vi "practice 4.vi"() -> ()   [LabVIEW 2018]
panel:
  out "文字列 8":string
  out "文字列 7":string
  out "数値 3":dbl
  in  "クラスタ":cluster{"数値":dbl, "数値 2":dbl}
  out "数値 2":dbl
  in  "文字列 6":string
  out "文字列 5":string
  in  "文字列 4":string
  out "文字列 3":string
  in  "文字列 2":string
  in  "文字列":string
  out "数値":dbl
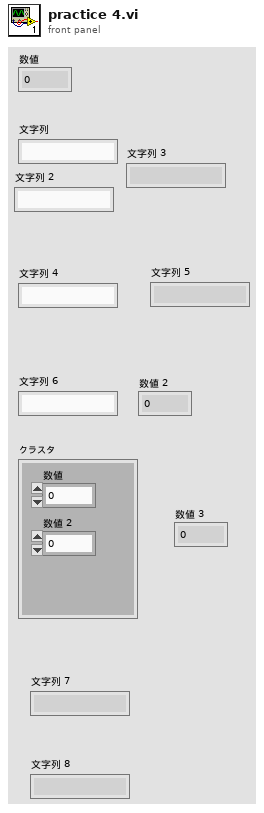
[diagram p1: front panel]
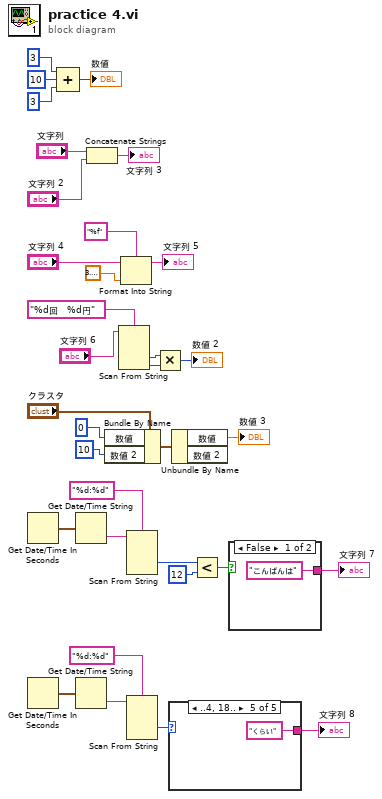
[diagram p0: block diagram]
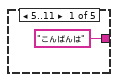
[diagram p2: hidden frame]
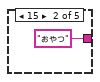
[diagram p3: hidden frame]
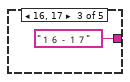
[diagram p4: hidden frame]
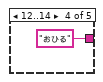
[diagram p5: hidden frame]
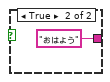
[diagram p6: hidden frame]
diagram:
  n1 = Get Date/Time In Seconds() -> (seconds since 1Jan1904=w12:timestamp)
  n2 = Get Date/Time In Seconds() -> (seconds since 1Jan1904=w3:timestamp)
  n3 = Compound Arithmetic op=unknown ("複合演算")(3, 10, 3) -> (→"数値":i32)
  n4 = Get Date/Time String(seconds (now)=w12) -> (time string=w6:string)  [unwired: 2 in, 1 out]
  n5 = Get Date/Time String(seconds (now)=w3) -> (time string=w5:string)  [unwired: 2 in, 1 out]
  n6 = Concatenate Strings("文字列", "文字列 2") -> (→"文字列 3":string)
  n7 = Bundle By Name(cluster="クラスタ", "数値"=0, "数値 2"=10) -> (w16:cluster{"数値":dbl, "数値 2":dbl})
  n8 = Scan From String(format string="%d回　%d円" ("形式文字列"), input string="文字列 6") -> (output 1=w20:i32, output 2=w19:i32)  [unwired: 4 in, 3 out]
  n9 = Format Into String(format string="%f", initial string="文字列 4", 3.141592653589793) -> (resulting string=→"文字列 5":string)  [unwired: 1 in, 1 out]
  n10 = Scan From String(format string="%d:%d", input string=w6) -> (output 1=w10:i32)  [unwired: 5 in, 3 out]
  n11 = Scan From String(format string="%d:%d", input string=w5) -> (output 1=w2:i32)  [unwired: 5 in, 3 out]
  n12 = Multiply(x=w20, y=w19) -> (x*y=→"数値 2":i32)
  n13 = case shown="..4, 18.." w2 {
    tunnel: ["こんばんは" "おやつ" "１６－１７" "おひる" "くらい"] -> w1
    frame 5..11 {
    }
    frame 15 {
    }
    frame 16, 17 {
    }
    frame 12..14 {
    }
    frame ..4, 18.. {
    }
  }
  "文字列 8" <- w1
  n14 = Unbundle By Name(w16) -> ("数値"=→"数値 3":dbl)  [unwired: 1 out]
  n15 = Less?(x=w10, y=12) -> (x < y?=w8:bool)
  n16 = case shown="FALSE" w8 {
    tunnel: ["こんばんは" "おはよう"] -> w7
    frame False {
    }
    frame True {
    }
  }
  "文字列 7" <- w7
